vi "XBEE send example.vi"() -> ()   [LabVIEW 2012]
panel:
  out "string sent":string
  in  "stop":bool
  out "String Received":string
  out "error out":errorcluster
  in  "String":string="$Hello World^"
  out "return count":u32
  in  "VISA resource name":refnum<visa-resource-name>="COM3"
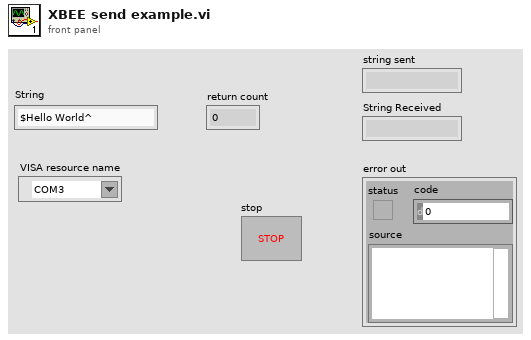
[diagram p1: front panel]
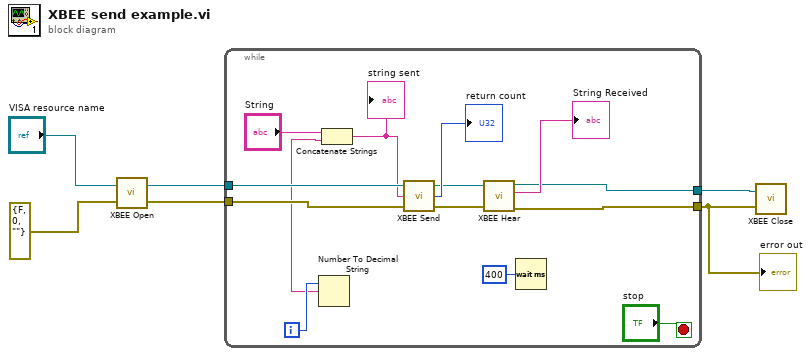
[diagram p0: block diagram]
diagram:
  n1 = call "XBEE Open.vi"("error in"=errorcluster {"status"=FALSE, "code"=0, "source"=""} ("error in (no error)"), "VISA resource name"="VISA resource name") -> ("error out"=w4:errorcluster, "VISA resource name out"=w5:refnum<visa-resource-name>)
  n2 = while {
    tunnel: w5 -> [w20]
    tunnel: w4 -> [w19]
    tunnel: [w14] -> w2
    tunnel: [w13] -> w1
    i -> [w9]
    stop <- "stop" stop-if-true
    n3 = Number To Decimal String(number=w9) -> (decimal integer string=w8:string)  [unwired: 1 in]
    n4 = Concatenate Strings("String", w8) -> (w7:string)
    "string sent" <- w7
    n5 = call "XBEE Send.vi"("error in (no error)"=w19, "String"=w7, "VISA resource name"=w20) -> ("error out"=w17:errorcluster, "return count"=→"return count":u32, "VISA resource name out"=w16:refnum<visa-resource-name>)
    n6 = call "XBEE Hear.vi"("VISA resource name"=w16, "error in (no error)"=w17) -> ("VISA resource name out"=w13:refnum<visa-resource-name>, "String Received"=→"String Received":string, "error out"=w14:errorcluster)  [unwired: 1 out]
    n7 = Wait (ms)(milliseconds to wait=u32 400) -> ()  [unwired: 1 out]
  }
  "error out" <- w2
  n8 = call "XBEE Close.vi"("error in (no error)"=w2, "VISA resource name"=w1) -> ()
